vi "Queue Driver LV2.vi"(0 "States[]":string[](array[string]), 2 "Name":string, 11 "Error In":errorcluster, 13 "Operation":T1=enum."Enqueue") -> (4 "Dequeued State":string, 15 "error out":errorcluster)   [LabVIEW 2021, in "Ball Launcher.lvlib"]
doc: "LV2 used for queue operations\nQueue used for enqueue/dequeue of States"
uses:
  Ball Launcher.lvlib
  Typedefs/Queue Operations.ctl
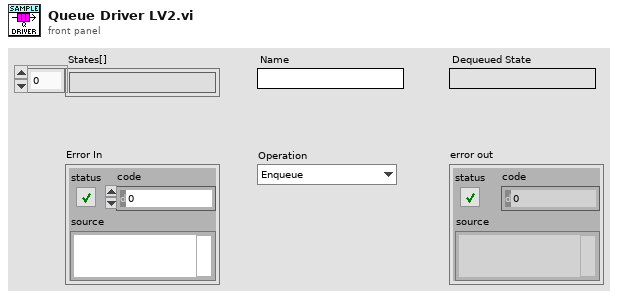
[diagram p1: front panel]
types:
  T1 = typedef "Ball Launcher.lvlib/Queue Operations.ctl" = enum16{"Create Q", "Enqueue", "Enstack", "Dequeue", "Flush Q", "Release Q"}
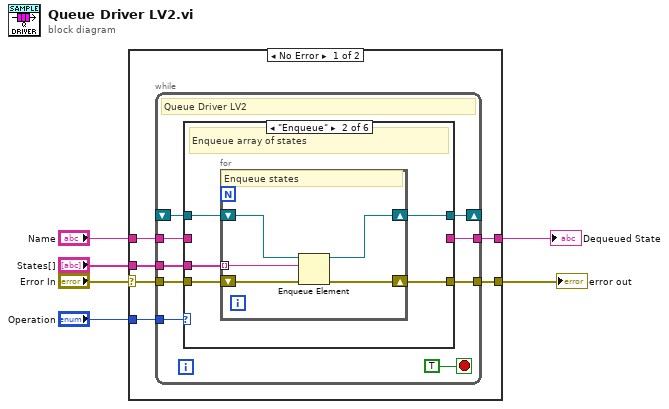
[diagram p0: block diagram]
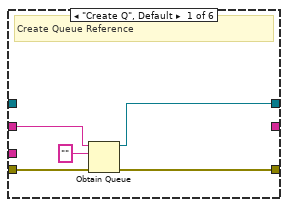
[diagram p2: hidden frame]
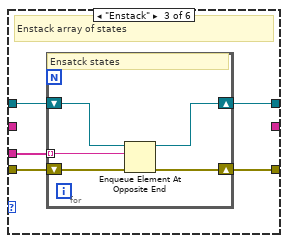
[diagram p3: hidden frame]
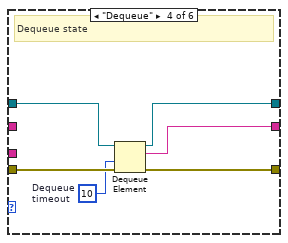
[diagram p4: hidden frame]
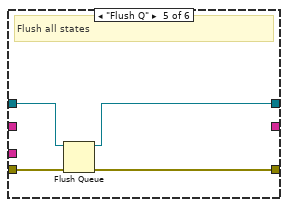
[diagram p5: hidden frame]
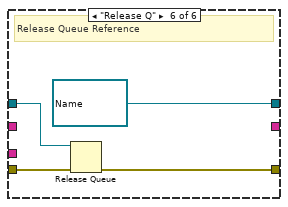
[diagram p6: hidden frame]
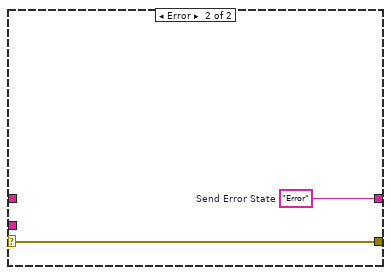
[diagram p7: hidden frame]
diagram:
  n1 = case shown="No Error" "Error In" {
    selector: "Error In" -> [w11 w62]
    tunnel: [w12 w62] -> w5
    tunnel: "Operation" -> [w10 _]
    tunnel: "Name" -> [w9 _]
    tunnel: "States[]" -> [w8 _]
    tunnel: [w7 w61] -> w1
    frame No Error {
      n2 = while {
        tunnel: [w21] -> w12
        tunnel: w11 -> [w20]
        tunnel: w10 -> [w19]
        tunnel: w9 -> [w16]
        tunnel: w8 -> [w15]
        shift-right: [w17] -> _
        shift-left: _ -> [w18]
        tunnel: [w14] -> w7
        stop <- TRUE stop-if-true
        # "Queue Driver LV2"
        n3 = case shown="\"Enqueue\"" w19 {
          tunnel: [w25 w31 w41 w52 w56 w60] -> w21
          tunnel: w20 -> [w26 w30 w40 w51 w55 w59]
          tunnel: w18 -> [_ w29 w39 w50 w54 w58]
          tunnel: [w22 w28 w38 w49 w53 refnum<queue> refnum ("queue out")] -> w17
          tunnel: w16 -> [w24 _ _ _ _ _]
          tunnel: w15 -> [_ w27 w37 _ _ _]
          tunnel: [_ _ _ w48 _ _] -> w14
          frame "Create Q", Default {
            # "Create Queue Reference"
            n4 = Obtain Queue(name (unnamed)=w24, element data type="" ("Name"), error in (no error)=w26) -> (queue out=w22:refnum<queue>, error out=w25:errorcluster)  [unwired: 2 in, 1 out]
          }
          frame "Enqueue" {
            # "Enqueue array of states"
            n5 = for {
              tunnel: w27 -> [w32] mode=indexing
              shift-right: [w36] -> w31
              shift-left: w30 -> [w35]
              shift-right: [w33] -> w28
              shift-left: w29 -> [w34]
              # "Enqueue states"
              n6 = Enqueue Element(queue=w34, element=w32, error in (no error)=w35) -> (queue out=w33:refnum<queue>, error out=w36:errorcluster)  [unwired: 1 in, 1 out]
            }
          }
          frame "Enstack" {
            # "Enstack array of states"
            n7 = for {
              tunnel: w37 -> [w42] mode=indexing
              shift-right: [w46] -> w41
              shift-left: w40 -> [w45]
              shift-right: [w43] -> w38
              shift-left: w39 -> [w44]
              # "Ensatck states"
              n8 = Enqueue Element At Opposite End(queue=w44, element=w42, error in (no error)=w45) -> (queue out=w43:refnum<queue>, error out=w46:errorcluster)  [unwired: 1 in, 1 out]
            }
          }
          frame "Dequeue" {
            w47 = 10  # Dequeue timeout
            # "Dequeue state"
            n9 = Dequeue Element(queue=w50, timeout in ms (-1)=w47, error in (no error)=w51) -> (queue out=w49:refnum<queue>, element=w48:string, error out=w52:errorcluster)  [unwired: 1 out]
          }
          frame "Flush Q" {
            # "Flush all states"
            n10 = Flush Queue(queue=w54, error in (no error)=w55) -> (queue out=w53:refnum<queue>, error out=w56:errorcluster)  [unwired: 1 out]
          }
          frame "Release Q" {
            # "Release Queue Reference"
            n11 = Release Queue(queue=w58, error in (no error)=w59) -> (error out=w60:errorcluster)  [unwired: 1 in, 2 out]
          }
        }
      }
    }
    frame Error {
      w61 = "Error"  # Send Error State
    }
  }
  "error out" <- w5
  "Dequeued State" <- w1
